vi "Log.vi"(8 "error in":errorcluster, 11 "File Path Control":path) -> (0 "error out":errorcluster, 3 "String 2":string)   [LabVIEW 2015]
panel:
  in  "stop":bool
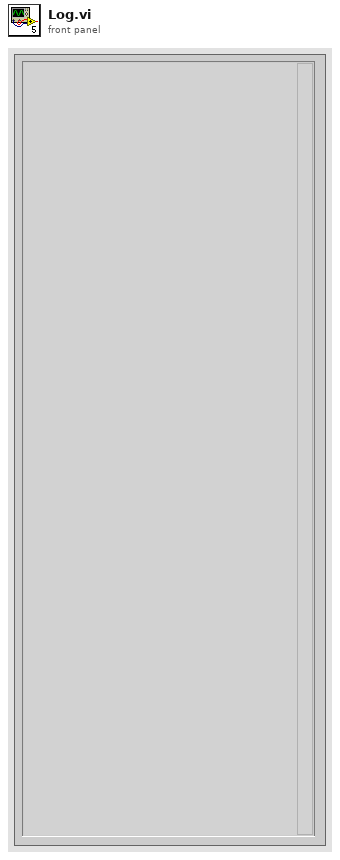
[diagram p1: front panel]
types:
  T1 = enum32{"Invalid", "Standard", "Closed", "Hidden", "Minimized", "Maximized"}
  T2 = enum16{"open", "replace", "create", "open or create", "replace or create", "replace or create with confirmation"}
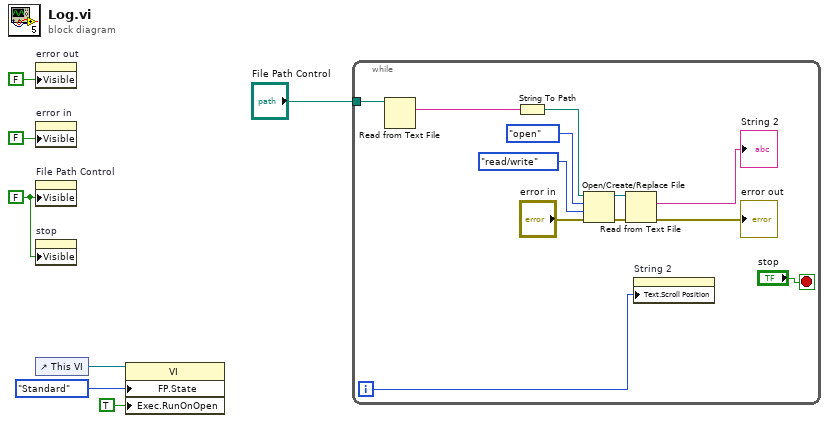
[diagram p0: block diagram]
diagram:
  w4 = FALSE ("Visible")
  n1 = property on="error out" class="Clust (strict)"("Visible"=FALSE) -> ()  [unwired: 2 in, 2 out]
  n2 = property on="error in" class="Clust (strict)"("Visible"=FALSE) -> ()  [unwired: 2 in, 2 out]
  n3 = property on="File Path Control" class="Path"("Visible"=w4) -> ()  [unwired: 2 in, 2 out]
  n4 = property on="stop" class="Bool"("Visible"=w4) -> ()  [unwired: 2 in, 2 out]
  n5 = control-ref of="This VI"() -> (w6:refnum<vi>)
  n6 = property class="VI"(reference=w6, "FP.State"=T1."Standard" ("Front Panel Window:State"), "Exec.RunOnOpen"=TRUE ("Execution:Run When Opened")) -> ()  [unwired: 1 in, 2 out]
  n7 = while {
    tunnel: "File Path Control" -> [w11]
    i -> [w8]
    stop <- "stop" stop-if-true
    n8 = Read from Text File(file (use dialog)=w11) -> (text=w13:string)  [unwired: 3 in, 3 out]
    n9 = String To Path(string=w13) -> (path=w12:path)
    n10 = Open/Create/Replace File(file path (use dialog)=w12, error in="error in", operation (0:open)=T2."open", access (0:read/write)=enum16{"read/write", "read-only", "write-only"}."read/write") -> (refnum out=w9:refnum<file>, error out=w10:errorcluster)  [unwired: 2 in, 1 out]
    n11 = Read from Text File(file (use dialog)=w9, error in=w10) -> (text=→"String 2":string, error out=→"error out":errorcluster)  [unwired: 2 in, 2 out]
    n12 = property on="String 2" class="Str"("Text.Scroll Position"=w8) -> ()  [unwired: 2 in, 2 out]
  }
